vi "Memory.Array.Numeric.DBL.New.vi"(7 "allocation limit (2^31: 2GiB)":u64=2147483647 format="%08x bytes", 8 "error in (no error)":errorcluster, 11 "number of elements":u64 format="%d elements") -> (0 "error out":errorcluster, 3 "DBL Array":refnum<class "Memory.Array.Numeric.DBL.lvclass">)   [LabVIEW 2016, in "Memory Manager.lvlib" / "Memory.Array.Numeric.DBL.lvclass"]
uses:
  Memory.Array.Numeric.DBL.lvclass
  C:/Users/Ryan/Documents/Git/Sourcetree/LabVIEW-Memory-Manager/Source/Library/Classes/Array/Array.Void/Memory.Array.Void.lvclass
  C:/Users/Ryan/Documents/Git/Sourcetree/LabVIEW-Memory-Manager/Source/Library/Classes/Array/Array.Numeric/Memory.Array.Numeric.lvclass
  Pointer/Pointer.Void/Memory.Pointer.Void.lvclass/Memory.Pointer.Void.ctl
  Array.Void/Memory.Array.Void.lvclass/Memory.Array.Void.ctl
  Array.Numeric/Memory.Array.Numeric.lvclass/Memory.Array.Numeric.ctl
  Array.Void/Methods/Memory.Array.Set Pointer.vi
  Array.Void/Methods/Memory.Array.Set Element Size.vi
  Array.Void/Methods/Memory.Array.Set Number of Elements.vi
  Pointer/Pointer.Void/Methods/Memory.Pointer.New.vi
  Pointer/Pointer.Void/Methods/Memory.Pointer.Allocate.vi
  Pointer/Pointer.Void/Methods/Memory.Pointer.Set Size.vi
  Pointer/Pointer.Void/Methods/Memory.Pointer.Set Address.vi
  Pointer/Pointer.Void/Methods/Memory.Pointer.Get Size.vi
  Pointer/Pointer.Void/Memory.Pointer.Void.lvclass
  Array.Numeric/Memory.Array.Numeric.lvclass
  Array.Void/Memory.Array.Void.lvclass
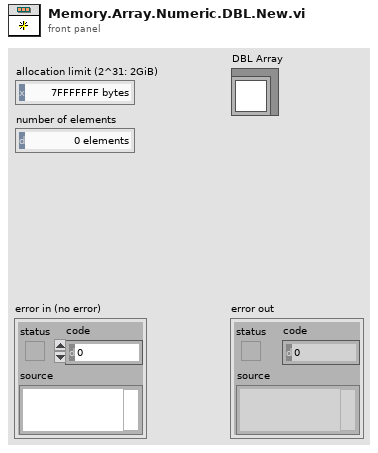
[diagram p1: front panel]
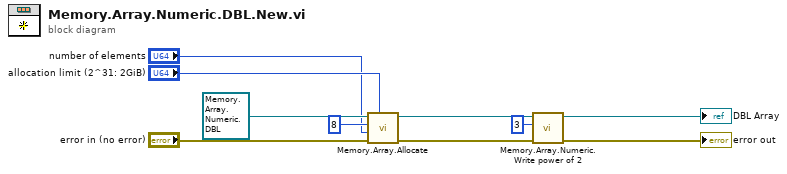
[diagram p0: block diagram]
diagram:
  n1 = call "Memory.Array.Allocate.vi"("allocation limit (2^31: 2GiB)"="allocation limit (2^31: 2GiB)", "error in (no error)"="error in (no error)", "number of elements"="number of elements", "size of element"=u64 8, "Array in"=refnum<class "Memory.Array.Numeric.DBL.lvclass"> refnum ("LabVIEW Memory Manager.lvlib:DBL Array")) -> ("error out"=w6:errorcluster, "Array out"=w8:refnum<class "Memory.Array.Numeric.DBL.lvclass">)  [unwired: 4 in, 1 out]
  n2 = call "Memory.Array.Numeric.Write power of 2.vi"("error in (no error)"=w6, "power of 2"=i16 3, "Numeric Array in"=w8) -> ("error out"=→"error out":errorcluster, "Numeric Array out"=→"DBL Array":refnum<class "Memory.Array.Numeric.DBL.lvclass">)  [unwired: 7 in]
